vi "GetScanAxis.vi"(1 "scan pair":T1) -> (2 "Axis 1":i32, 3 "Axis 2":i32, 4 "Axis 3":i32)   [LabVIEW 2022 SP3]
uses:
  Motion Controllers/-MotionRoutines/ScanAxis.ctl
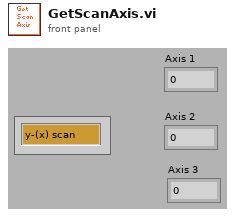
[diagram p1: front panel]
types:
  T1 = typedef "ScanAxis.ctl" = enum16{"y-(x) scan", "x-(y) scan", "z-(x) scan", "z-(y) scan", "y-(z) scan", "x-(z) scan", "w-(x) scan", "w-(y) scan", "w-(z) scan", "x-(w) scan", "y-(w) scan", "z-(w) scan"}
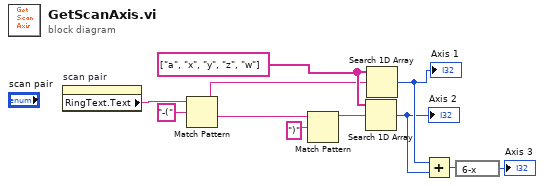
[diagram p0: block diagram]
diagram:
  w9 = string[] ["a", "x", "y", "z", "w"]
  n1 = property on="scan pair" class="Enum (strict)"() -> ("RingText.Text"=w11:string)  [unwired: 2 in, 2 out]
  n2 = Match Pattern(string=w11, regular expression="-(") -> (before substring=w8:string, after substring=w7:string)  [unwired: 3 out]
  n3 = Match Pattern(string=w7, regular expression=")") -> (before substring=w10:string)  [unwired: 4 out]
  n4 = Search 1D Array(1D array=w9, element=w10) -> (index of element=w3:i32)  [unwired: 1 out]
  "Axis 2" <- w3
  n5 = Search 1D Array(1D array=w9, element=w8) -> (index of element=w4:i32)  [unwired: 1 out]
  "Axis 1" <- w4
  n6 = Add(x=w4, y=w3) -> (x+y=w2:i32)
  n7 = expression code="6-x"(w2) -> (→"Axis 3":i32)
